vi "Read configuration.vi"(8 "error in":errorcluster, 11 "PLTarget PC in":refnum<class "PLTarget PC.lvclass">) -> (0 "error out":errorcluster, 2 "configuration":refnum<class "NISE_CEF_serializable configuration.lvclass">, 3 "PLTarget PC out":refnum<class "PLTarget PC.lvclass">)   [LabVIEW 2013, in "PLTarget PC.lvclass"]
uses:
  PLTarget PC.lvclass
  <vilib>/NI/Configuration Framework/serializable configuration/NISE_CEF_serializable configuration.lvclass
  PLTarget PC.lvclass/PLTarget PC.ctl
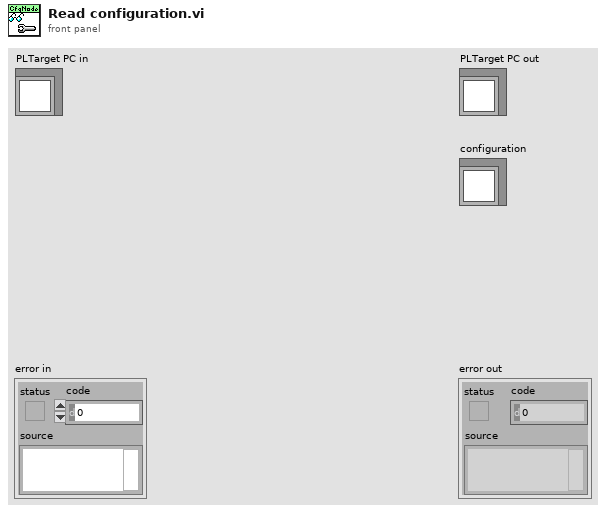
[diagram p1: front panel]
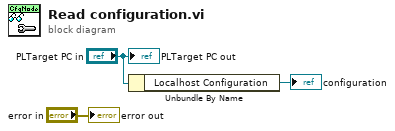
[diagram p0: block diagram]
diagram:
  n1 = Unbundle By Name("PLTarget PC in") -> ("Localhost Configuration"=→"configuration":refnum<class "PL_Target Configuration.lvclass">)
  "error out" <- "error in"
  "PLTarget PC out" <- "PLTarget PC in"
